vi "UpdateShake.vi"(8 "error in (no error)":errorcluster, 11 "TilesLoopData in":T1) -> (0 "error out":errorcluster, 3 "TilesLoopData out":T1)   [LabVIEW 2019, in "RT_Game.lvlib" / "Engine.lvclass"]
uses:
  Engine.lvclass
  TilesLoopData.ctl
  Coordinate.ctl
  SlideJob.ctl
  ScreenSide.ctl
  FPGA_Interface.ctl
  <vilib>/Utility/error.llb/Error Cluster From Error Code.vi
  <vilib>/rvi/errors/niLvFpgaAdjustHostInterfaceError.vi
  <vilib>/rvi/interface/nirviReadWriteControl/nirviReadWriteControl.xnode
  FPGA Bitfiles/myriogameconsole_FPGATarget_Main_ntsPRcBZGxk.lvbitx
  NiFpgaLv.dll
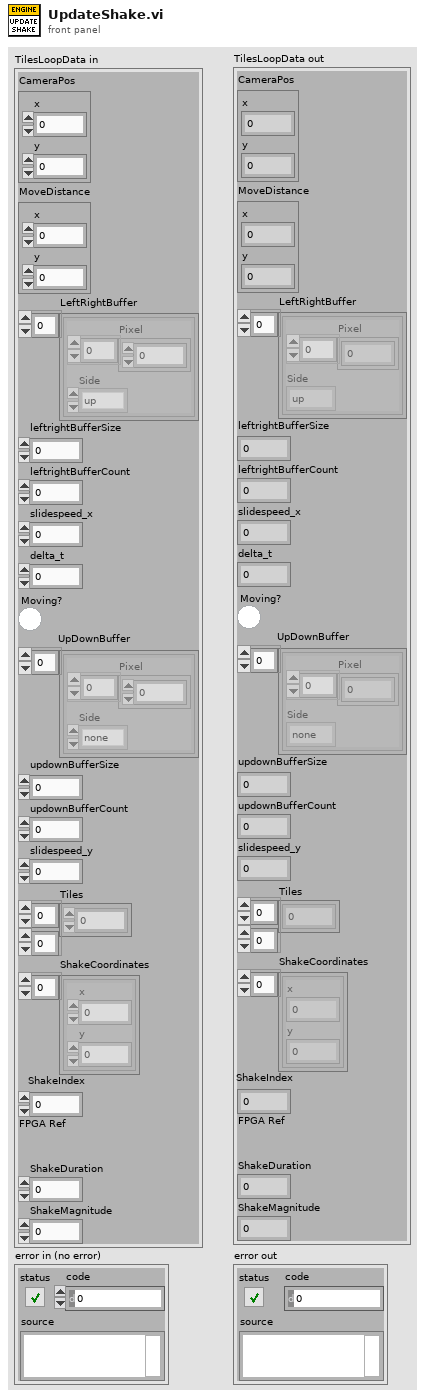
[diagram p1: front panel]
types:
  T1 = typedef "RT_Game.lvlib/Engine.lvclass/TilesLoopData.ctl" = cluster{"CameraPos":T2, "MoveDistance":T2, "LeftRightBuffer":T3[], "leftrightBufferSize":i16, "leftrightBufferCount":i16, "slidespeed_x":dbl, "delta_t":dbl, "Moving?":bool, "UpDownBuffer":T3[], "updownBufferSize":i16, "updownBufferCount":i16, "slidespeed_y":dbl, "Tiles":u32[][], "ShakeCoordinates":T2[], "ShakeIndex":i16, "FPGA Ref":T5, "ShakeDuration":dbl, "ShakeMagnitude":dbl}
  T2 = typedef "RT_Game.lvlib/Engine.lvclass/Coordinate.ctl" = cluster{"x":dbl, "y":dbl}
  T3 = typedef "RT_Game.lvlib/Engine.lvclass/SlideJob.ctl" = cluster{"Pixel":u32[], "Side":T4}
  T4 = typedef "RT_Game.lvlib/Engine.lvclass/ScreenSide.ctl" = enum16{"up", "down", "left", "right", "none"}
  T5 = typedef "FPGA_Interface.ctl" = refnum<k20>
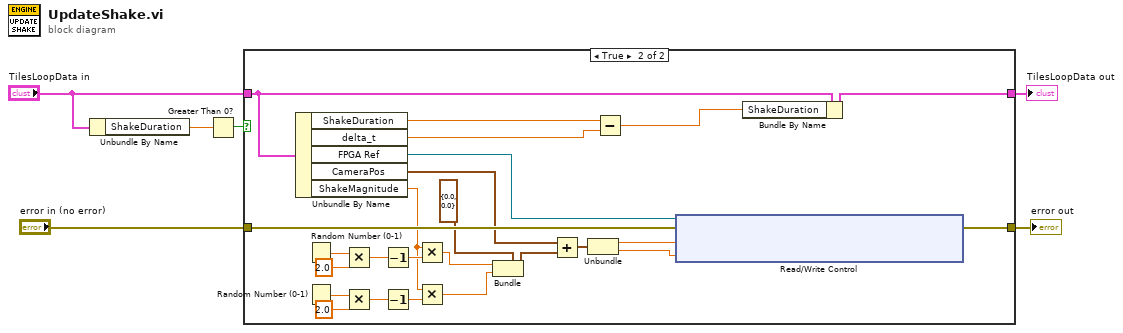
[diagram p0: block diagram]
diagram:
  n1 = Unbundle By Name("TilesLoopData in") -> ("ShakeDuration"=w4:dbl)
  n2 = Greater Than 0?(x=w4) -> (x > 0?=w1:bool)
  n3 = case shown="True" w1 {
    tunnel: "TilesLoopData in" -> [w8 w33]
    tunnel: [w8 w12] -> w5
    tunnel: "error in (no error)" -> [w7 w32]
    tunnel: [w7 w31] -> w2
    frame False {
    }
    frame True {
      n4 = Unbundle By Name(w33) -> ("ShakeDuration"=w11:dbl, "delta_t"=w9:dbl, "FPGA Ref"=w30:T5, "CameraPos"=w29:T2, "ShakeMagnitude"=w14:dbl)
      n5 = Random Number (0-1)() -> (number: 0 to 1=w23:dbl)
      n6 = Random Number (0-1)() -> (number: 0 to 1=w15:dbl)
      n7 = Multiply(x=w23, y=2.0) -> (x*y=w21:dbl)
      n8 = Multiply(x=w15, y=2.0) -> (x*y=w17:dbl)
      n9 = Decrement(x=w21) -> (x-1=w20:dbl)
      n10 = Decrement(x=w17) -> (x-1=w18:dbl)
      n11 = Multiply(x=w14, y=w20) -> (x*y=w19:dbl)
      n12 = Multiply(x=w14, y=w18) -> (x*y=w13:dbl)
      n13 = Bundle(cluster=T2 {"x"=0.0, "y"=0.0} ("y"), "x"=w19, "y"=w13) -> (w24:T2)
      n14 = Add(x=w29, y=w24) -> (x+y=w28:T2)
      n15 = Unbundle(w28) -> ("x"=w27:dbl, "y"=w26:dbl)
      n16 = Subtract(x=w11, y=w9) -> (x-y=w10:dbl)
      n17 = xnode "Read/Write Control"("FPGA VI Reference In"=w30, "error in"=w32, "x_Shift"=w27, "y_Shift"=w26) -> ("error out"=w31:errorcluster)  [unwired: 1 out]
      n18 = Bundle By Name(cluster=w33, "ShakeDuration"=w10) -> (w12:T1)
    }
  }
  "error out" <- w2
  "TilesLoopData out" <- w5
